vi "Update.vi"(8 "error in (no error)":errorcluster, 11 "LINX-SN3218 in":refnum<class "LINX-SN3218.lvclass">) -> (0 "error out":errorcluster, 3 "LINX-SN3218 out":refnum<class "LINX-SN3218.lvclass">)   [LabVIEW 2020, in "LINX-SN3218.lvclass"]
doc: "Low-level VI to trigger an output update. This is called automatically by the Set Channel PWM function."
uses:
  LINX-SN3218.lvclass
  LINX I2C/LINX I2C.lvclass
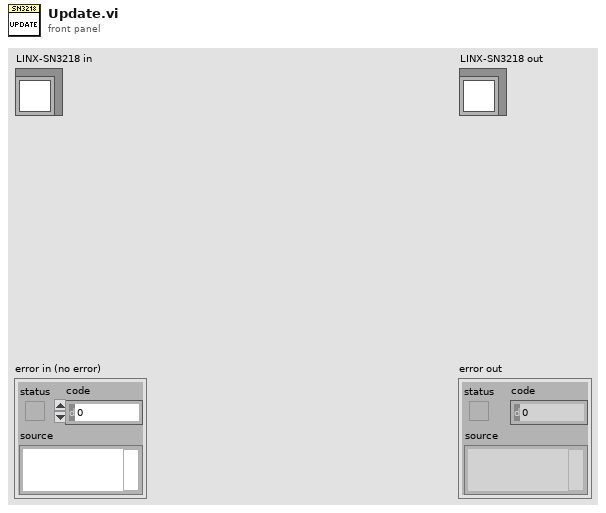
[diagram p1: front panel]
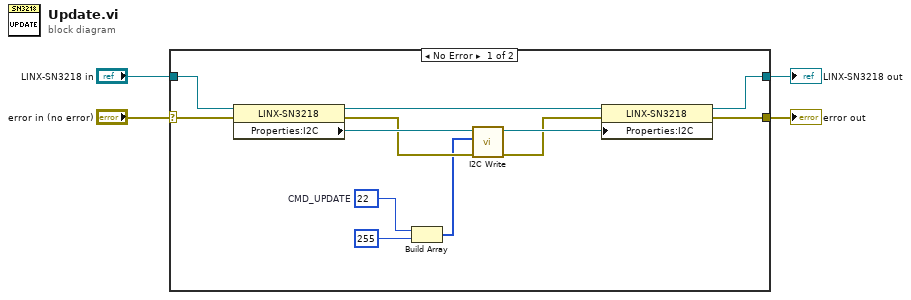
[diagram p0: block diagram]
diagram:
  n1 = case shown="No Error" "error in (no error)" {
    selector: "error in (no error)" -> [w14 w18]
    tunnel: [w8 w18] -> w3
    tunnel: [w12 w17] -> w1
    tunnel: "LINX-SN3218 in" -> [w16 w17]
    frame No Error {
      w7 = u8 22  # CMD_UPDATE
      n2 = property class="LINX-SN3218"(reference=w16, error in=w14) -> (reference out=w13:refnum<class "LINX-SN3218.lvclass">, error out=w10:errorcluster, "Properties:I2C"=w15:refnum<class "LINX I2C.lvclass">)
      n3 = Build Array(w7, u8 255) -> (w6:u8[])
      n4 = call "I2C Write.vi"("error in (no error)"=w10, "Bytes to Write"=w6, "LINX I2C in"=w15) -> ("error out"=w9:errorcluster, "LINX I2C out"=w11:refnum<class "LINX I2C.lvclass">)  [unwired: 7 in]
      n5 = property class="LINX-SN3218"(reference=w13, error in=w9, "Properties:I2C"=w11) -> (reference out=w12:refnum<class "LINX-SN3218.lvclass">, error out=w8:errorcluster)
    }
    frame Error {
    }
  }
  "error out" <- w3
  "LINX-SN3218 out" <- w1
